vi "Chirp_FPGA_prototype.vi"(8 "Iteration":fxp<+/-,64,32>, 9 "Chirp/Fft Pair 1 - Chirp Rate":fxp<+/-,64,2>=0.005545560037717223, 10 "Imaginary In":fxp<+/-,64,2>, 11 "Real In":fxp<+/-,64,2>) -> (2 "Imaginary Out":fxp<+/-,64,2>, 3 "Real Out":fxp<+/-,64,2>)   [LabVIEW 2015]
uses:
  <vilib>/rvi/FXPMathLib/FxpDiv/subVIs/nifxpmath_Div_SimConfig.ctl
  <vilib>/rvi/FXPMathLib/FxpSinAndCos/subVIs/nifxpmath_SinAndCos_SimConfig.ctl
  <vilib>/rvi/FXPMathLib/FxpDiv/simVIs/DllFxpDivTemp_sub.vi
  <vilib>/rvi/FXPMathLib/FxpSinAndCos/simVIs/DllFxpSinAndCosTemp_sub.vi
  <vilib>/rvi/FXPMathLib/FxpReciprocal/XNode/nifxpmath_Reciprocal.xnode
  <vilib>/rvi/FXPMathLib/FxpDiv/XNode/nifxpmath_Div.xnode
  <vilib>/rvi/FXPMathLib/FxpMul/XNode/nifxpmath_Multiplier.xnode
  <vilib>/rvi/FXPMathLib/FxpSub/XNode/nifxpmath_Sub.xnode
  <vilib>/rvi/FXPMathLib/FxpSinAndCos/XNode/nifxpmath_SinAndCos.xnode
  <vilib>/rvi/FXPMathLib/FxpAdd/XNode/nifxpmath_Add.xnode
  <vilib>/rvi/FXPMathLib/sim/FxpSim.dll
panel:
  out "ang":fxp<+/-,64,32>
  out "time":fxp<+/-,64,32>
  out "c":fxp<+/-,64,2>=0.99993896484375
  out "d":fxp<+/-,64,2>=-0.0126953125
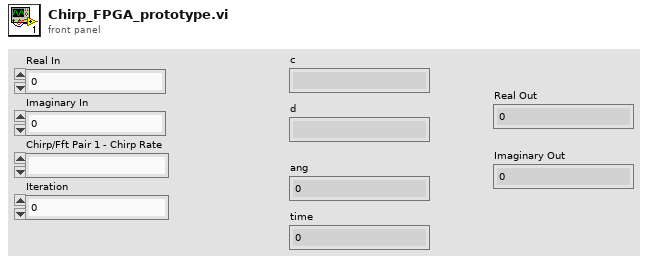
[diagram p1: front panel]
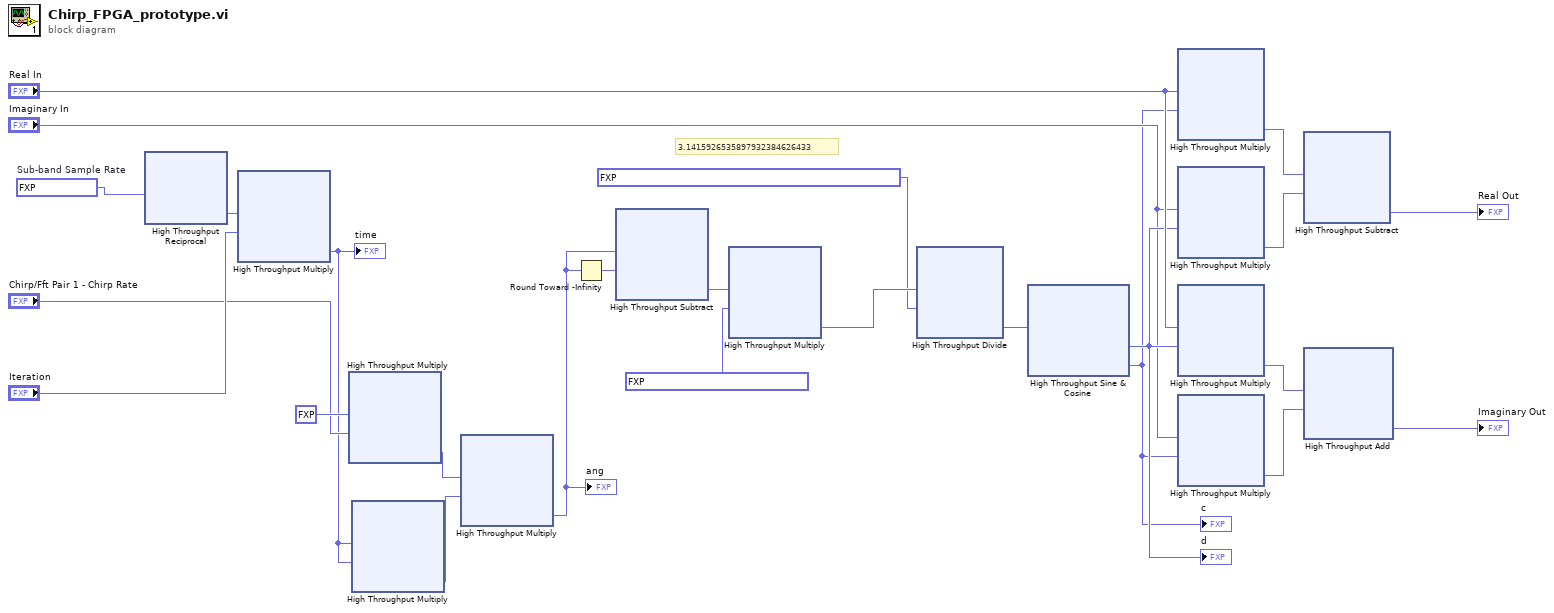
[diagram p0: block diagram]
diagram:
  w22 = fxp<+,64,32> 9765.62109375  # Sub-band Sample Rate
  # "3.1415926535897932384626433"
  n1 = xnode "High Throughput Reciprocal"("x"=w22) -> ("1/x"=w21:fxp<+,64,32>)
  n2 = xnode "High Throughput Multiply"("x"=w21, "y"="Iteration") -> ("x*y"=w16:fxp<+/-,64,32>)
  "time" <- w16
  n3 = xnode "High Throughput Multiply"("x"=fxp<+,1,0> 0.5 ("value"), "y"="Chirp/Fft Pair 1 - Chirp Rate") -> ("x*y"=w20:fxp<+/-,64,32>)
  n4 = xnode "High Throughput Multiply"("x"=w16, "y"=w16) -> ("x*y"=w19:fxp<+/-,64,32>)
  n5 = xnode "High Throughput Multiply"("x"=w20, "y"=w19) -> ("x*y"=w15:fxp<+/-,64,32>)
  "ang" <- w15
  n6 = Round Toward -Infinity(1:w15) -> (0:w14:fxp<+/-,32,32>)
  n7 = xnode "High Throughput Subtract"("x"=w15, "y"=w14) -> ("x-y"=w24:fxp<+/-,64,33>)
  n8 = xnode "High Throughput Multiply"("x"=w24, "y"=fxp<+/-,32,4> 6.2831853069365025) -> ("x*y"=w3:fxp<+/-,64,32>)
  n9 = xnode "High Throughput Divide"("x"=w3, "y"=fxp<+,64,3> dbl? 1.8937212861877052e+176) -> ("x/y"=w1:fxp<+/-,64,4>)
  n10 = xnode "High Throughput Sine & Cosine"("x (pi)"=w1) -> ("sin(x)"=w8:fxp<+/-,64,2>, "cos(x)"=w4:fxp<+/-,64,2>)
  "c" <- w4
  "d" <- w8
  n11 = xnode "High Throughput Multiply"("x"="Real In", "y"=w4) -> ("x*y"=w13:fxp<+/-,64,2>)
  n12 = xnode "High Throughput Multiply"("x"="Imaginary In", "y"=w8) -> ("x*y"=w12:fxp<+/-,64,2>)
  n13 = xnode "High Throughput Multiply"("x"="Real In", "y"=w8) -> ("x*y"=w11:fxp<+/-,64,4>)
  n14 = xnode "High Throughput Multiply"("x"="Imaginary In", "y"=w4) -> ("x*y"=w10:fxp<+/-,64,4>)
  n15 = xnode "High Throughput Subtract"("x"=w13, "y"=w12) -> ("x-y"=→"Real Out":fxp<+/-,64,2>)
  n16 = xnode "High Throughput Add"("x"=w11, "y"=w10) -> ("x+y"=→"Imaginary Out":fxp<+/-,64,2>)
